vi "Completed_var.vi"() -> ()   [LabVIEW 2019]
panel:
  in  "Completed":bool
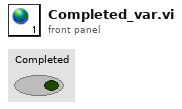
[diagram p1: front panel]
diagram:
